vi "Module Next ID.vi"(8 "error in (no error)":errorcluster, 11 "Increment? (T)":bool=TRUE) -> (0 "error out":errorcluster, 2 "Next ID":i32, 3 "ID SEQ":refnum<queue>)   [LabVIEW 2022 SP3, in "Core.lvlib"]
uses:
  Core.lvlib
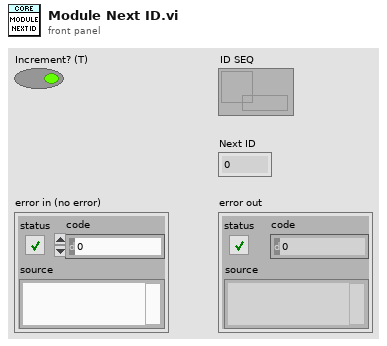
[diagram p1: front panel]
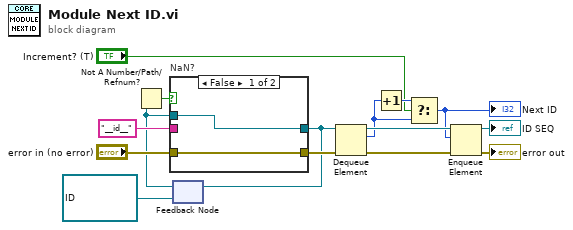
[diagram p0: block diagram]
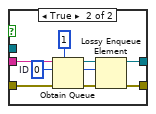
[diagram p2: hidden frame]
diagram:
  n1 = feedback #1(refnum<queue> refnum ("queue out")) -> (w12:refnum<queue>)
  n2 = Not A Number/Path/Refnum?(number/path/refnum=w12) -> (NaN/Path/Refnum?=w11:bool)
  n3 = case "NaN?" shown="False" w11 {
    tunnel: "__id__" ("name (unnamed)") -> [_ w24]
    tunnel: [w17 w22] -> w9
    tunnel: [w16 w19] -> w14
    tunnel: "error in (no error)" -> [w16 w18]
    tunnel: w12 -> [w17 _]
    frame False {
    }
    frame True {
      w20 = 0  # ID
      n4 = Obtain Queue(max queue size (-1, unlimited)=1, name (unnamed)=w24, element data type=w20, error in (no error)=w18) -> (queue out=w23:refnum<queue>, error out=w21:errorcluster)  [unwired: 1 in, 1 out]
      n5 = Lossy Enqueue Element(queue=w23, element=w20, error in (no error)=w21) -> (queue out=w22:refnum<queue>, error out=w19:errorcluster)  [unwired: 2 out]
    }
  }
  n6 = feedback-in #1(w9) -> ()
  n7 = Dequeue Element(queue=w9, error in (no error)=w14) -> (queue out=w5:refnum<queue>, element=w3:i32, error out=w6:errorcluster)  [unwired: 1 in, 1 out]
  n8 = Increment(x=w3) -> (x+1=w4:i32)
  n9 = Select(t=w4, s="Increment? (T)", f=w3) -> (s? t:f=w2:i32)
  "Next ID" <- w2
  n10 = Enqueue Element(queue=w5, element=w2, error in (no error)=w6) -> (queue out=→"ID SEQ":refnum<queue>, error out=→"error out":errorcluster)  [unwired: 1 in, 1 out]
